vi "case according to command.vi"(8 "error in":errorcluster, 11 "command":T1=22 items=["NO_Action", "start", "pause", "resum", "stop", "config"]) -> (0 "error out":errorcluster, 2 "case":string="Command - Wkf_control")   [LabVIEW 2015]
uses:
  controls.llb/command.ctl
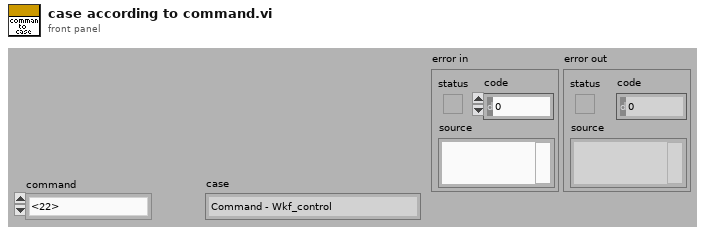
[diagram p1: front panel]
types:
  T1 = typedef "command.ctl" = u16
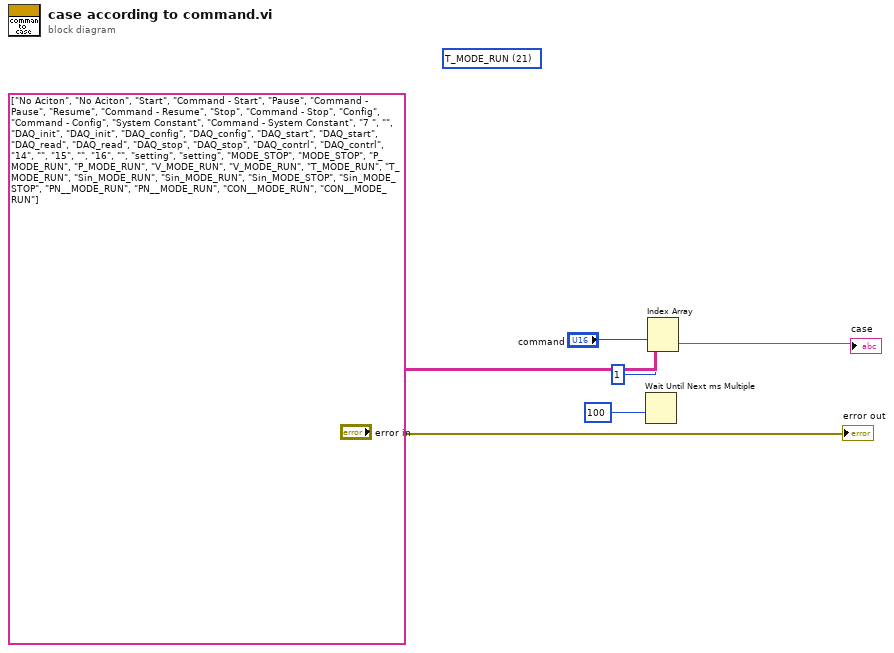
[diagram p0: block diagram]
diagram:
  (unwired) T1 21 items=["NO_Action", "start", "pause", "resum", "stop", "config", "System_constant", "7", "DAQ_init", "DAQ_config", "DAQ_start", "DAQ_read", "DAQ_stop", "DAQ_contrl", "14", "15", "16", "setting", "MODE_STOP", "P_MODE_RUN", "V_MODE_RUN", "T_MODE_RUN"] ("command")
  n1 = Wait Until Next ms Multiple(millisecond multiple=u32 100) -> ()  [unwired: 1 out]
  n2 = Index Array(array=string[][] [["No Aciton", "No Aciton"], ["Start", "Command - Start"], ["Pause", "Command - Pause"], ["Resume", "Command - Resume"], ["Stop", "Command - Stop"], ["Config", "Command - Config"], ["System Constant", "Command - System Constant"], ["7 ", ""], ["DAQ_init", "DAQ_init"], ["DAQ_config", "DAQ_config"], ["DAQ_start", "DAQ_start"], ["DAQ_read", "DAQ_read"], ["DAQ_stop", "DAQ_stop"], ["DAQ_contrl", "DAQ_contrl"], ["14", ""], ["15", ""], ["16", ""], ["setting", "setting"], ["MODE_STOP", "MODE_STOP"], ["P_MODE_RUN", "P_MODE_RUN"], ["V_MODE_RUN", "V_MODE_RUN"], ["T_MODE_RUN", "T_MODE_RUN"], ["Sin_MODE_RUN", "Sin_MODE_RUN"], ["Sin_MODE_STOP", "Sin_MODE_STOP"], ["PN__MODE_RUN", "PN__MODE_RUN"], ["CON__MODE_RUN", "CON__MODE_RUN"]] ("command to case"), index (row)="command", index (col)=1 ("disabled index (col)")) -> (element=→"case":string)
  "error out" <- "error in"
